vi "Unit 5M.vi"() -> ()   [LabVIEW 2023]
panel:
  out "isTrue":bool=TRUE
  in  "Мащаб 1 сек:1":u32=1000
  in  "k Минути":dbl format="%#_2g"
  out "∆Nk %":dbl format="%#_3g"
  out "Минути":dbl format="%#_2g"
  out "Час":i64
  out "tmp":dbl
  out "Часа":dbl format="%#_2g"
  out "Минути":dbl format="%#_4g"
  out "dN %/мин":dbl format="%#_2g"
  in  "dN/dT %/ h":dbl format="%#_2g"
  in  "N1 %":dbl format="%#_3g"
  out "Waveform Chart":T1(graph)
  out "N след 1 минута":dbl format="%#_3g"
  out "N текуща %":dbl format="%#_3g"
  in  "N2 %":dbl format="%#_3g"
  # "със"
  # "За"
  # "min"
  # "мил. сек."
  # "след"
  # "Общо време"
  # ":"
  # "="
  # "%"
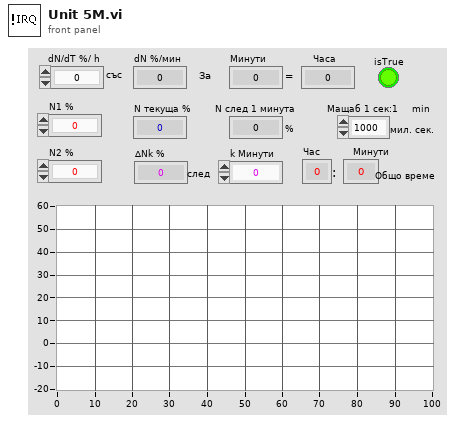
[diagram p1: front panel]
types:
  T1 = cluster{"N текуща % ":dbl, "N2 % ":dbl, "Nк %  ":dbl}
  T2 = cluster{"N текуща % ":dbl, "N2 % ":dbl, "∆Nk %  ":dbl}
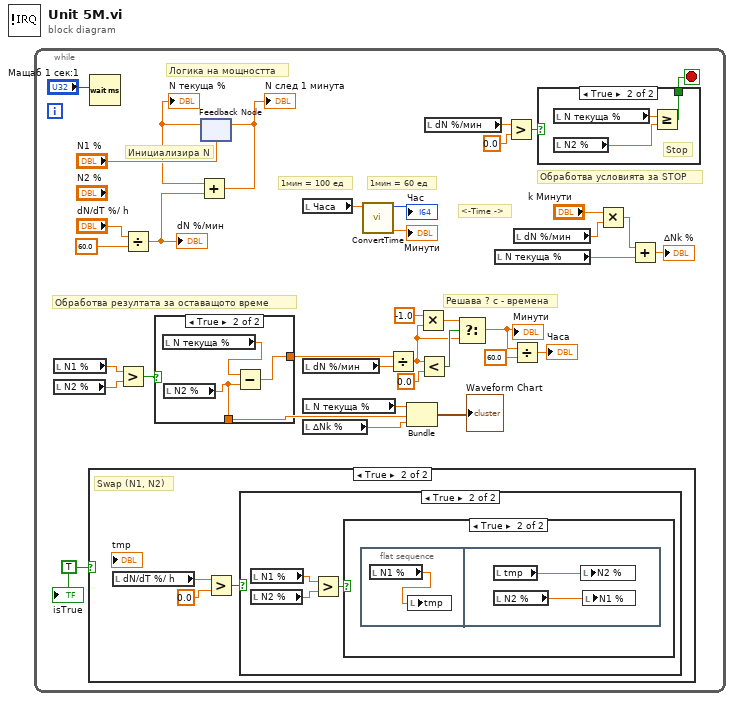
[diagram p0: block diagram]
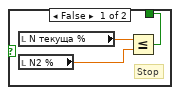
[diagram p2: hidden frame]
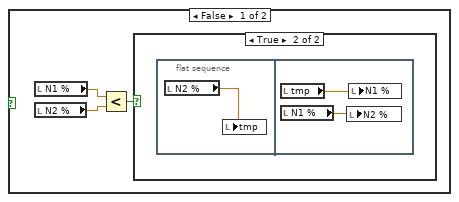
[diagram p4: hidden frame]
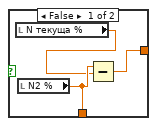
[diagram p7: hidden frame]
diagram:
  n1 = while {
    stop <- w1 stop-if-true
    w21 = TRUE
    # "1мин = 60 ед"
    # "1мин = 100 ед"
    # "Решава ? с - времена"
    # "<-Time ->"
    # "Обработва резултата за оставащото време"
    # "Обработва условията за STOP"
    # "Логика на мощността"
    # "Инициализира N"
    n2 = local read "N1 %"() -> (w30:dbl)
    n3 = local read "N2 %"() -> (w29:dbl)
    n4 = case shown="True" w21 {
      frame False {
      }
      frame True {
        # "Swap (N1, N2)"
        n5 = local read "dN/dT %/ h"() -> (w46:dbl)
        n6 = Greater?(x=w46, y=0.0) -> (0:w44:bool)
        n7 = case shown="True" w44 {
          frame False {
            n8 = local read "N1 %"() -> (w49:dbl)
            n9 = local read "N2 %"() -> (w48:dbl)
            n10 = Less?(x=w49, y=w48) -> (x < y?=w47:bool)
            n11 = case shown="True" w47 {
              frame False {
              }
              frame True {
                n12 = flat-sequence {
                  frame #0 {
                    n13 = local read "N2 %"() -> (w50:dbl)
                    n14 = local write "tmp"(w50) -> ()
                  }
                  frame #1 {
                    n15 = local read "tmp"() -> (w51:dbl)
                    n16 = local read "N1 %"() -> (w52:dbl)
                    n17 = local write "N2 %"(w52) -> ()
                    n18 = local write "N1 %"(w51) -> ()
                  }
                }
              }
            }
          }
          frame True {
            n19 = local read "N1 %"() -> (w55:dbl)
            n20 = local read "N2 %"() -> (w54:dbl)
            n21 = Greater?(x=w55, y=w54) -> (0:w53:bool)
            n22 = case shown="True" w53 {
              frame False {
              }
              frame True {
                n23 = flat-sequence {
                  frame #0 {
                    n24 = local read "N1 %"() -> (w56:dbl)
                    n25 = local write "tmp"(w56) -> ()
                  }
                  frame #1 {
                    n26 = local read "tmp"() -> (w58:dbl)
                    n27 = local read "N2 %"() -> (w57:dbl)
                    n28 = local write "N2 %"(w58) -> ()
                    n29 = local write "N1 %"(w57) -> ()
                  }
                }
              }
            }
          }
        }
      }
    }
    n30 = Wait (ms)(milliseconds to wait="Мащаб 1 сек:1") -> ()  [unwired: 1 out]
    n31 = Greater?(x=w30, y=w29) -> (0:w28:bool)
    n32 = Divide(x="dN/dT %/ h", y=60.0) -> (x/y=w34:dbl)
    "dN %/мин" <- w34
    n33 = case shown="True" w28 {
      tunnel: [w61 w64] -> w27
      tunnel: [w60 w62] -> w24
      frame False {
        n34 = local read "N текуща %"() -> (w59:dbl)
        n35 = local read "N2 %"() -> (w60:dbl)
        n36 = Subtract(x=w60, y=w59) -> (x-y=w61:dbl)
      }
      frame True {
        n37 = local read "N текуща %"() -> (w63:dbl)
        n38 = local read "N2 %"() -> (w62:dbl)
        n39 = Subtract(x=w63, y=w62) -> (x-y=w64:dbl)
      }
    }
    n40 = feedback #1("N1 %") -> (w33:dbl)
    "N текуща %" <- w33
    n41 = Add(x=w33, y=w34) -> (x+y=w32:dbl)
    "N след 1 минута" <- w32
    n42 = feedback-in #1(w32) -> ()
    n43 = local read "Часа"() -> (w20:dbl)
    n44 = local read "dN %/мин"() -> (w17:dbl)
    n45 = local read "N текуща %"() -> (w25:dbl)
    n46 = local read "∆Nk %"() -> (w2:dbl)
    n47 = call "ConvertTime.vi"("Час1"=w20) -> ("Минути"=→"Минути":dbl, "Час"=→"Час":i64)  [unwired: 9 in]
    n48 = Divide(x=w27, y=w17) -> (x/y=w11:dbl)
    n49 = Bundle("N текуща %"=w25, "N2 %"=w24, "∆Nk %"=w2) -> (→"Waveform Chart":T2)  [unwired: 1 in]
    n50 = Multiply(x=-1.0 ("y"), y=w11) -> (x*y=w14:dbl)
    n51 = Less?(x=w11, y=0.0) -> (x < y?=w15:bool)
    n52 = local read "dN %/мин"() -> (w5:dbl)
    n53 = Select(t=w14, s=w15, f=w11) -> (s? t:f=w13:dbl)
    "Минути" <- w13
    n54 = local read "N текуща %"() -> (w6:dbl)
    n55 = Greater?(x=w5, y=0.0) -> (0:w3:bool)
    n56 = Divide(x=w13, y=60.0) -> (x/y=→"Часа":dbl)
    n57 = local read "dN %/мин"() -> (w9:dbl)
    n58 = case shown="True" w3 {
      tunnel: [w40 w41] -> w1
      frame False {
        # "Stop"
        n59 = local read "N текуща %"() -> (w39:dbl)
        n60 = local read "N2 %"() -> (w38:dbl)
        n61 = Less Or Equal?(x=w39, y=w38) -> (x <= y?=w40:bool)
      }
      frame True {
        # "Stop"
        n62 = local read "N текуща %"() -> (w43:dbl)
        n63 = local read "N2 %"() -> (w42:dbl)
        n64 = Greater Or Equal?(x=w43, y=w42) -> (x >= y?=w41:bool)
      }
    }
    n65 = Multiply(x="k Минути", y=w9) -> (x*y=w7:dbl)
    n66 = Add(x=w7, y=w6) -> (x+y=→"∆Nk %":dbl)
    "isTrue" <- w21
  }
